vi "SPCWriteSETforSPC.vi"(5 "ActiveModule":string[](array[string]), 6 "NoOfRoutingChannels":u32=1, 7 "mode":i32=1, 8 "ErrorIn":errorcluster, 9 "SPCdata":T1={"base_adr"=52672, "init"=0, "cfd_limit_low"=-0.0, "cfd_limit_high"=5.019608, "cfd_zc_level"=-5.2913384, "cfd_holdoff"=5.0, "sync_zc_level"=-5.2913384, "sync_holdoff"=4.0, "sync_threshold"=-70.588234, "tac_range"=50.033573, "sync_freq_div"=1, "tac_gain"=1, "tac_offset"=5.098039, "tac_limit_low"=0.0, "tac_limit_high"=100.0, "adc_resolution"=12, "ext_latch_delay"=0, "collect_time"=1.0, "display_time"=1.0, "repeat_time"=10.0, "stop_on_time"=1, "stop_on_ovfl"=1, "dither_range"=128, "count_incr"=1, "mem_bank"=0, "dead_time_comp"=0, "scan_control"=0, "routing_mode"=0, "tac_enable_hold"=0.0, "pci_card_no"=-1, "mode"=5, "scan_size_x"=1, "scan_size_y"=1, "scan_rout_x"=1, "scan_rout_y"=1, "scan_flyback"=65537, "scan_borders"=0, "scan_polarity"=0, "pixel_clock"=1, "line_compression"=1, "trigger"=0, "pixel_time"=1e-07, "ext_pixclk_div"=1, "rate_count_time"=1.0, "macro_time_clk"=0, "add_select"=0, "test_eep"=1, "adc_zoom"=0, "img_size_x"=1, "img_size_y"=1, "img_rout_x"=1, "img_rout_y"=1, "xy_gain"=1, "master_clock"=0, "adc_sample_delay"=0, "detector_type"=1, "chan_enable"=4191231, "chan_slope"=0, "chan_spec_no"=34835, "tdc_control"=0, "tdc_offset1"=0.0, "tdc_offset2"=0.0, "tdc_offset3"=0.0, "tdc_offset4"=0.0, "future_reserve1"=0, "future_reserve2"=0, "future_reserve3"=0, "future_reserve4"=0, "future_reserve5"=0, "future_reserve6"=0, "future_reserve7"=0} {"scan_flyback" format="%x"}, 10 "SP_MODE":i32=7, 11 "SET-FilePath":path) -> (0 "ErrorOut":errorcluster)   [LabVIEW 2019]
doc: "This VI demonstrates how a SET-file as pair for a corresponding SPC-file can be generated and written to disc.\n<b>Note:</b> In order to be readable by Spcm.exe SPC-files need to be accompanied by a corresponding SET-file. \nFor a description of the *.set file format see: SPC_data_file_structure.h\n\ninfo@becker-hickl.com"
uses:
  SPC_Controls/bhfile_header.ctl
  SPC_Controls/FileType.ctl
  SPC_Controls/BHModuleType.ctl
  SPC_Controls/SPCdata.ctl
panel:
  out "BHModuleType":T2=43 format="x%x" items=["SPC-130"=32, "SPC-600"=33, "SPC-630"=34, "SPC-700"=35, "SPC-730"=36, "SPC-830"=37, "SPC-140"=38, "SPC-930"=39, "SPC-150"=40, "DPC-230"=41, "SPC-130EM"=42, "SPC-160"=43, "SPC-150N"=46, "SPC-150NX"=128, "SPC-160X"=129, "SPC-160PCIE"=130, "SPC-130EMN"=131, "SPC-180N"=132, "SPC-180NX"=133, "SPC-180NXX"=134, "SPC-180N-USB"=135, "SPC-130IN"=136, "SPC-130INX"=137, "SPC-130INXX"=138, "SPC-QC-104"=139, "Simulation"=-1]
  out "bhfile_header":T3 {"chksum" format="x%x"; "header_valid" format="x%x"}
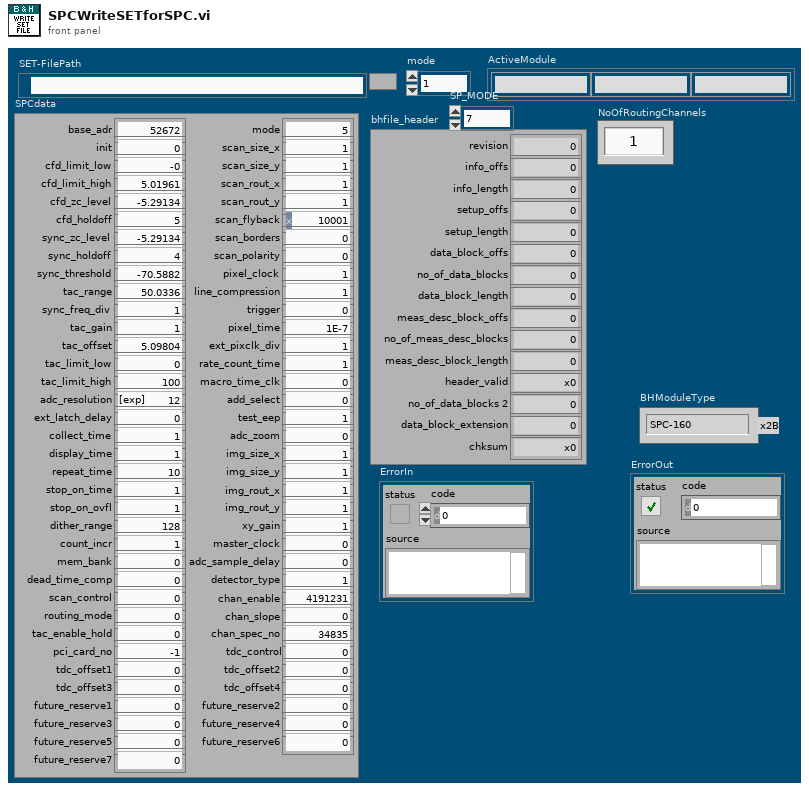
[diagram p1: front panel]
types:
  T1 = typedef "SPCdata.ctl" = cluster{"base_adr":u16, "init":i16, "cfd_limit_low":sgl, "cfd_limit_high":sgl, "cfd_zc_level":sgl, "cfd_holdoff":sgl, "sync_zc_level":sgl, "sync_holdoff":sgl, "sync_threshold":sgl, "tac_range":sgl, "sync_freq_div":i16, "tac_gain":i16, "tac_offset":sgl, "tac_limit_low":sgl, "tac_limit_high":sgl, "adc_resolution":i16, "ext_latch_delay":i16, "collect_time":sgl, "display_time":sgl, "repeat_time":sgl, "stop_on_time":i16, "stop_on_ovfl":i16, "dither_range":i16, "count_incr":i16, "mem_bank":i16, "dead_time_comp":i16, "scan_control":u16, "routing_mode":u16, "tac_enable_hold":sgl, "pci_card_no":i16, "mode":u16, "scan_size_x":u32, "scan_size_y":u32, "scan_rout_x":u32, "scan_rout_y":u32, "scan_flyback":u32, "scan_borders":u32, "scan_polarity":u16, "pixel_clock":u16, "line_compression":u16, "trigger":u16, "pixel_time":sgl, "ext_pixclk_div":u32, "rate_count_time":sgl, "macro_time_clk":i16, "add_select":i16, "test_eep":i16, "adc_zoom":i16, "img_size_x":u32, "img_size_y":u32, "img_rout_x":u32, "img_rout_y":u32, "xy_gain":i16, "master_clock":i16, "adc_sample_delay":i16, "detector_type":i16, "chan_enable":u32, "chan_slope":u32, "chan_spec_no":u32, "tdc_control":u32, "tdc_offset1":sgl, "tdc_offset2":sgl, "tdc_offset3":sgl, "tdc_offset4":sgl, "future_reserve1":u64, "future_reserve2":u64, "future_reserve3":u64, "future_reserve4":u64, "future_reserve5":u64, "future_reserve6":u64, "future_reserve7":u64}
  T2 = typedef "BHModuleType.ctl" = i16
  T3 = typedef "bhfile_header.ctl" = cluster{"revision":i16, "info_offs":i32, "info_length":i16, "setup_offs":i32, "setup_length":u16, "data_block_offs":i32, "no_of_data_blocks":i16, "data_block_length":u32, "meas_desc_block_offs":i32, "no_of_meas_desc_blocks":i16, "meas_desc_block_length":i16, "header_valid":u16, "no_of_data_blocks 2":u32, "data_block_extension":u16, "chksum":u16}
  T4 = typedef "FileType.ctl" = u16
  T5 = enum16{"open", "replace", "create", "open or create", "replace or create", "replace or create with confirmation"}
  T6 = enum16{"big-endian, network order", "native, host order", "little-endian"}
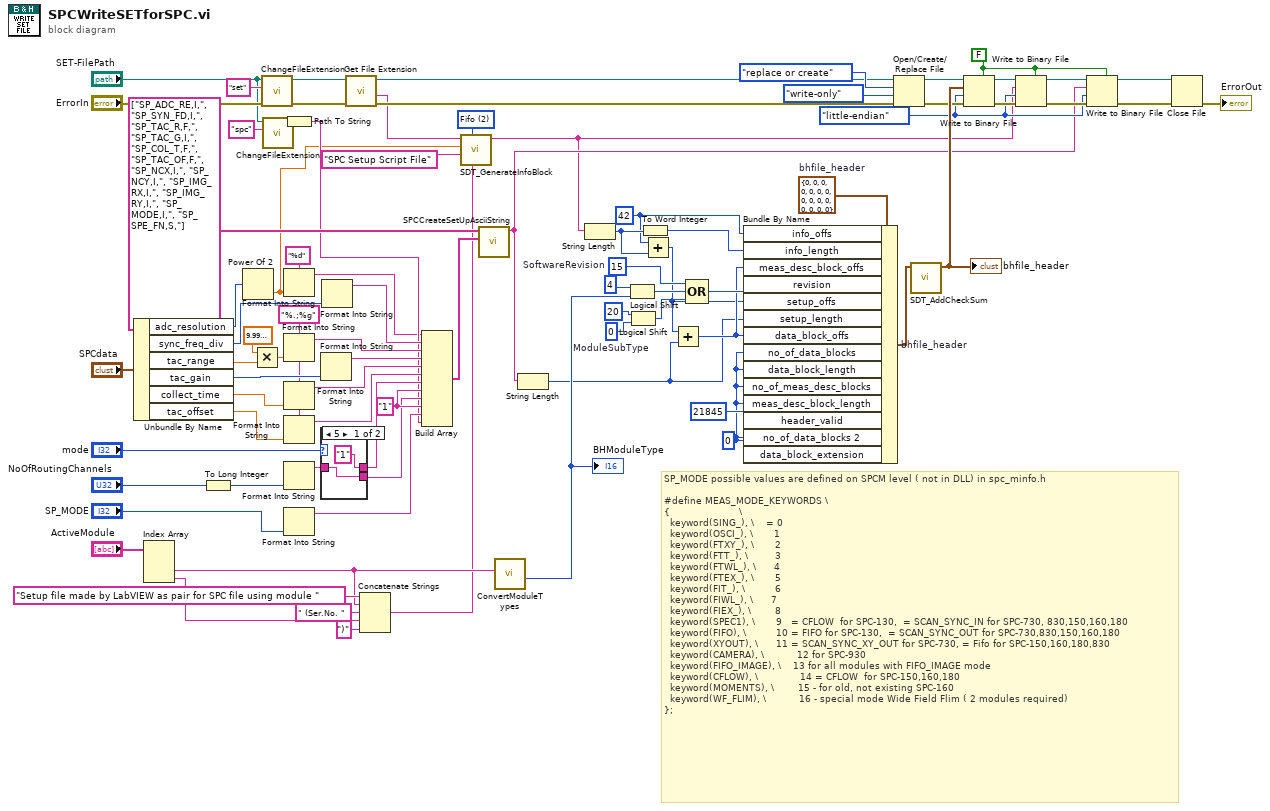
[diagram p0: block diagram]
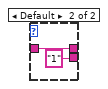
[diagram p2: hidden frame]
diagram:
  w2 = T4 2 items=["non-Fifo"=1, "Fifo"=2, "FifoImage"=3] ("FileType")
  w3 = T3 {"revision"=0, "info_offs"=0, "info_length"=0, "setup_offs"=0, "setup_length"=0, "data_block_offs"=0, "no_of_data_blocks"=0, "data_block_length"=0, "meas_desc_block_offs"=0, "no_of_meas_desc_blocks"=0, "meas_desc_block_length"=0, "header_valid"=0, "no_of_data_blocks 2"=0, "data_block_extension"=0, "chksum"=0}  # bhfile_header
  w6 = 42 ("Info Offset")
  w42 = "%.;%g" ("format string")
  w43 = "1" ("element")
  w70 = i16 0  # ModuleSubType
  w75 = i16 15  # SoftwareRevision
  w34 = u16 0 ("data_block_extension")
  w59 = FALSE ("prepend array or string size? (T)")
  w58 = T6."little-endian" ("byte order (0:big-endian, network order)")
  # "SP_MODE possible values are defined on SPCM level ( not in DLL) in spc_minfo.h\n\n#define MEAS_MODE_KEYWORDS \\\n{                       \\\n  keyword(SING_), \\    = 0\n  keyword(OSCI_), \\       1\n  keyword(FTXY_), \\       2\n  keyword(FTT_), \\         3\n  keyword(FTWL_), \\      4\n  keyword(FTEX_), \\       5\n  keyword(FIT_), \\          6\n  keyword(FIWL_), \\      7 \n  keyword(FIEX_), \\        8\n  keyword(SPEC1), \\       9   = CFLOW  for SPC-130,  = SCAN_SYNC_IN for SPC-730, 830,150,160,180\n  keyword(FIFO), \\          10 = FIFO for SPC-130,  = SCAN_SYNC_OUT for SPC-730,830,150,160,180\n  keyword(XYOUT), \\      11 = SCAN_SYNC_XY_OUT for SPC-730, = Fifo for SPC-150,160,180,830\n  keyword(CAMERA), \\           12 for SPC-930\n  keyword(FIFO_IMAGE), \\    13 for all modules with FIFO_IMAGE mode\n  keyword(CFLOW), \\              14 = CFLOW  for SPC-150,160,180\n  keyword(MOMENTS), \\        15 - for old, not existing SPC-160\n  keyword(WF_FLIM), \\           16 - special mode Wide Field Flim ( 2 modules required)\n};"
  n1 = Unbundle By Name("SPCdata") -> ("adc_resolution"=w11:i16, "sync_freq_div"=w54:i16, "tac_range"=w61:sgl, "tac_gain"=w48:i16, "collect_time"=w47:sgl, "tac_offset"=w45:sgl)
  n2 = Index Array(array="ActiveModule") -> (element #2=w18:string, element #3=w16:string)  [unwired: 3 in, 1 out]
  n3 = To Long Integer(number="NoOfRoutingChannels") -> (32bit integer=w35:i32)
  n4 = Power Of 2(x=w11) -> (2^x=w1:dbl)
  n5 = Multiply(x=sgl 1e-09 ("y"), y=w61) -> (x*y=w51:sgl)
  n6 = call "ChangeFileExtension.vi"("ErrorIn"="ErrorIn", "NewExtension"="set", "OldPath"="SET-FilePath") -> ("ErrorOut"=w24:errorcluster, "NewPath"=w26:path)  [unwired: 7 in]
  n7 = call "ChangeFileExtension.vi"("NewExtension"="spc", "OldPath"="SET-FilePath") -> ("NewPath"=w21:path)  [unwired: 8 in, 1 out]
  n8 = Path To String(path=w21) -> (string=w20:string)
  n9 = Format Into String(format string="%d", w1) -> (resulting string=w14:string)  [unwired: 2 in, 1 out]
  n10 = Format Into String(format string=w42, w51) -> (resulting string=w50:string)  [unwired: 2 in, 1 out]
  n11 = Format Into String(format string=w42, w47) -> (resulting string=w46:string)  [unwired: 2 in, 1 out]
  n12 = Format Into String(format string=w42, w45) -> (resulting string=w44:string)  [unwired: 2 in, 1 out]
  n13 = Format Into String(w35) -> (resulting string=w40:string)  [unwired: 3 in, 1 out]
  n14 = Format Into String("SP_MODE") -> (resulting string=w32:string)  [unwired: 3 in, 1 out]
  n15 = Format Into String(w48) -> (resulting string=w49:string)  [unwired: 3 in, 1 out]
  n16 = case shown="5" "mode" {
    tunnel: w40 -> [w85 w87]
    tunnel: ["1" w87] -> w39
    tunnel: [w85 "1"] -> w38
    frame 5 {
    }
    frame Default {
    }
  }
  n17 = Format Into String(w54) -> (resulting string=w53:string)  [unwired: 3 in, 1 out]
  n18 = call <vilib>:"Get File Extension.vi"("error in (no error)"=w24, "file"=w26) -> ("error out"=w68:errorcluster, "filename without extension"=w12:string, "dup file"=w28:path)  [unwired: 5 in, 2 out]
  n19 = Concatenate Strings("Setup file made by LabVIEW as pair for SPC file using module " ("Contents"), w18, " (Ser.No. " ("string"), w16, ")" ("string")) -> (w10:string)
  n20 = Build Array(w14, w53, w50, w49, w46, w44, w39, w43, w38, w43, w32, w20) -> (w52:string[])
  n21 = call "SDT_GenerateInfoBlock.vi"("Contents"=w10, "FileType"=w2, "FileID"="SPC Setup Script File" ("IDENTIFICATION"), "adc_re[dig]"=w1, "FilenameNoExtension"=w12) -> ("Info Block"=w7:string)  [unwired: 6 in]
  n22 = call "SPCCreateSetUpAsciiString.vi"("Value"=w52, "Key"=string[] ["SP_ADC_RE,I,", "SP_SYN_FD,I,", "SP_TAC_R,F,", "SP_TAC_G,I,", "SP_COL_T,F,", "SP_TAC_OF,F,", "SP_NCX,I,", "SP_NCY,I,", "SP_IMG_RX,I,", "SP_IMG_RY,I,", "SP_MODE,I,", "SP_SPE_FN,S,"]) -> ("SetUpAsciiString"=w29:string)  [unwired: 9 in]
  n23 = call "ConvertModuleTypes.vi"("ModuleTypeStringIn"=w18) -> ("BHModuleType"=w63:T2)  [unwired: 8 in, 2 out]
  "BHModuleType" <- w63
  n24 = String Length(string=w29) -> (length=w30:i32)
  n25 = String Length(string=w7) -> (length=w8:i32)
  n26 = Logical Shift(y=i16 4, x=w63) -> (x << y=w74:T2)
  n27 = Logical Shift(y=i16 20, x=w70) -> (x << y=w71:i16)
  n28 = To Word Integer(number=w8) -> (16bit integer=w5:i16)
  n29 = Add(x=w6, y=w8) -> (x+y=w4:i32)
  n30 = Add(x=w4, y=w30) -> (x+y=w31:i32)
  n31 = Compound Arithmetic op=OR(w75, w74, w71) -> (w73:T2)
  n32 = Bundle By Name "bhfile_header"(cluster=w3, "info_offs"=w6, "info_length"=w5, "meas_desc_block_offs"=w31, "revision"=w73, "setup_offs"=w4, "setup_length"=w30, "data_block_offs"=w31, "no_of_data_blocks"=w34, "data_block_length"=w34, "no_of_meas_desc_blocks"=w34, "meas_desc_block_length"=w34, "header_valid"=u16 21845, "no_of_data_blocks 2"=w34, "data_block_extension"=w34) -> (w78:T3)
  n33 = Open/Create/Replace File(file path (use dialog)=w28, error in=w68, operation (0:open)=T5."replace or create", access (0:read/write)=enum16{"read/write", "read-only", "write-only"}."write-only") -> (refnum out=w81:refnum<file>, error out=w67:errorcluster)  [unwired: 2 in, 1 out]
  n34 = call "SDT_AddCheckSum.vi"("bhfile_header"=w78) -> ("HeaderWithChkSum"=w77:T3)  [unwired: 9 in, 1 out]
  "bhfile_header" <- w77
  n35 = Write to Binary File(file (use dialog)=w81, data=w77, error in=w67, 5:w59, 9:w58) -> (refnum out=w80:refnum<file>, error out=w66:errorcluster)  [unwired: 1 in, 1 out]
  n36 = Write to Binary File(file (use dialog)=w80, data=w7, error in=w66, 5:w59, 9:w58) -> (refnum out=w69:refnum<file>, error out=w65:errorcluster)  [unwired: 1 in, 1 out]
  n37 = Write to Binary File(file (use dialog)=w69, data=w29, error in=w65, 5:w59, 9:w58) -> (refnum out=w36:refnum<file>, error out=w37:errorcluster)  [unwired: 1 in, 1 out]
  n38 = Close File(refnum=w36, error in=w37) -> (error out=→"ErrorOut":errorcluster)  [unwired: 1 out]
